vi "Test Config Iface Readback String.vi"(8 "error in (no error)":errorcluster, 11 "Test Case In":refnum<class "Configuration Interface Test.lvclass">) -> (0 "error out":errorcluster, 3 "Test Case Out":refnum<class "Configuration Interface Test.lvclass">)   [LabVIEW 2020, in "Configuration Interface Test.lvclass"]
uses:
  Configuration Interface Test.lvclass
  Framework/Configuration/Configuration.lvclass
  <vilib>/Asteme/LUnit/Test Case.lvclass
  C:/Program Files (x86)/National Instruments/LabVIEW 2020/vi.lib/Asteme/LUnit/Test Case.lvclass
  C:/Users/anton/Documents/GitHub/Triarc-Framework/source/Framework Test/Configuration Interface Test/Configuration Interface Test.lvclass
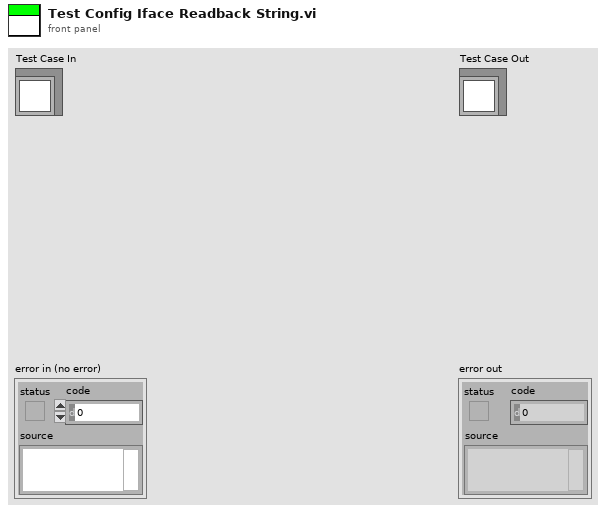
[diagram p1: front panel]
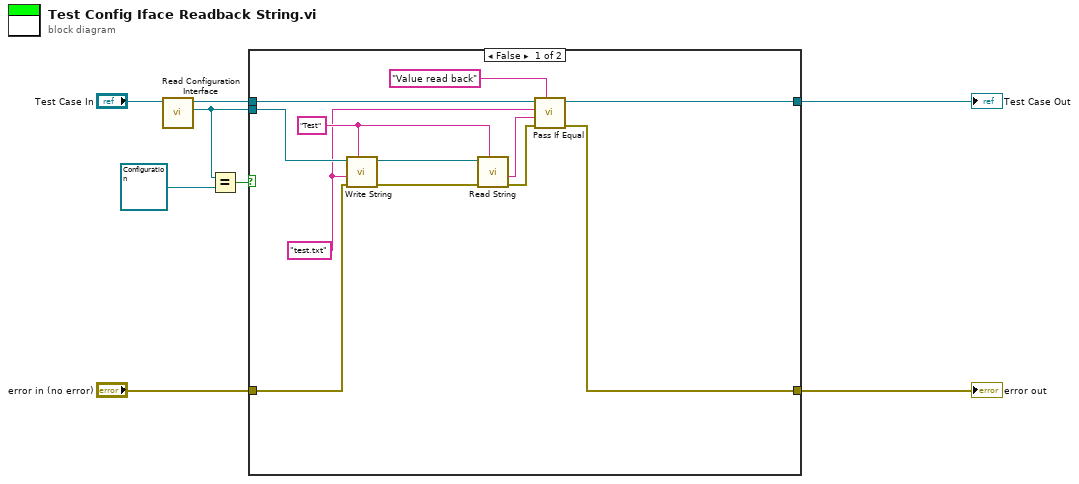
[diagram p0: block diagram]
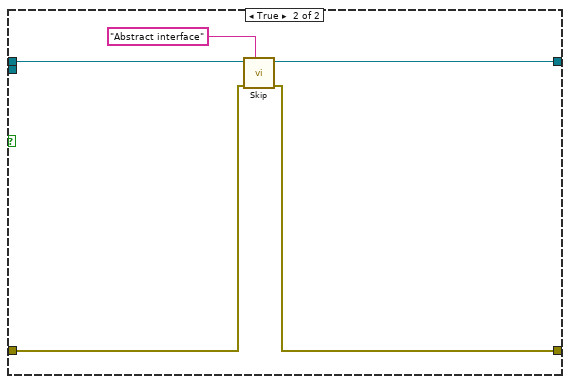
[diagram p2: hidden frame]
diagram:
  n1 = call "Read Configuration Interface.vi"("Configuration Interface Test In"="Test Case In") -> ("Configuration"=w3:refnum<class "Configuration.lvclass">, "Configuration Interface Test Out"=w6:refnum<class "Configuration Interface Test.lvclass">)  [unwired: 9 in]
  n2 = Equal?(x=w3, y=refnum<class "Configuration.lvclass"> refnum ("Configuration")) -> (x = y?=w1:bool)
  n3 = case shown="False" w1 {
    tunnel: [w17 w22] -> w7
    tunnel: w6 -> [w16 w25]
    tunnel: [w15 w24] -> w5
    tunnel: "error in (no error)" -> [w10 w23]
    tunnel: w3 -> [w13 _]
    frame False {
      w9 = "test.txt"
      w18 = "Test" ("key")
      n4 = call-dynamic "Write String.vi"("key"=w18, "error in (no error)"=w10, "value"=w9, "Configuration File In"=w13) -> ("error out"=w19:errorcluster, "Configuration File Out"=w20:refnum<class "Configuration.lvclass">)  [unwired: 6 in]
      n5 = call-dynamic "Read String.vi"("key"=w18, "error in (no error)"=w19, "Configuration File In"=w20) -> ("error out"=w14:errorcluster, "value"=w11:string)  [unwired: 6 in, 1 out]
      n6 = call <vilib>:"Pass If Equal.vi"("Description"="Value read back", "error in (no error)"=w14, "Actual"=w11, "Expected"=w9, "Test Case In"=w16) -> ("error out"=w17:errorcluster, "Test Case Out"=w15:refnum<class "Configuration Interface Test.lvclass">)  [unwired: 5 in]
    }
    frame True {
      n7 = call <vilib>:"Skip.vi"("Description"="Abstract interface", "error in (no error)"=w23, "Test Case In"=w25) -> ("error out"=w22:errorcluster, "Test Case Out"=w24:refnum<class "Configuration Interface Test.lvclass">)  [unwired: 7 in]
    }
  }
  "error out" <- w7
  "Test Case Out" <- w5
